vi "Send.vi"(8 "error in (no error)":errorcluster, 10 "Message":refnum<class "BaseMessage.lvclass">, 11 "StringReader in":refnum<class "StringReader.lvclass">) -> (0 "error out":errorcluster, 2 "Sent message":refnum<class "BaseMessage.lvclass">, 3 "StringReader out":refnum<class "StringReader.lvclass">)   [LabVIEW 2013, in "StringReader.lvclass"]
doc: "Send a message to the remote destination"
uses:
  StringReader.lvclass
  Message/BaseMessage/BaseMessage.lvclass
  BaseReader/BaseReader.lvclass
  <vilib>/Utility/error.llb/whitespace.ctl
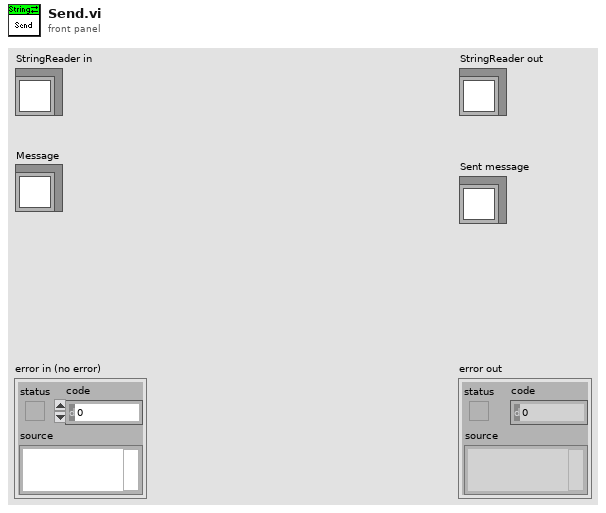
[diagram p1: front panel]
types:
  T1 = typedef "whitespace.ctl" = u16
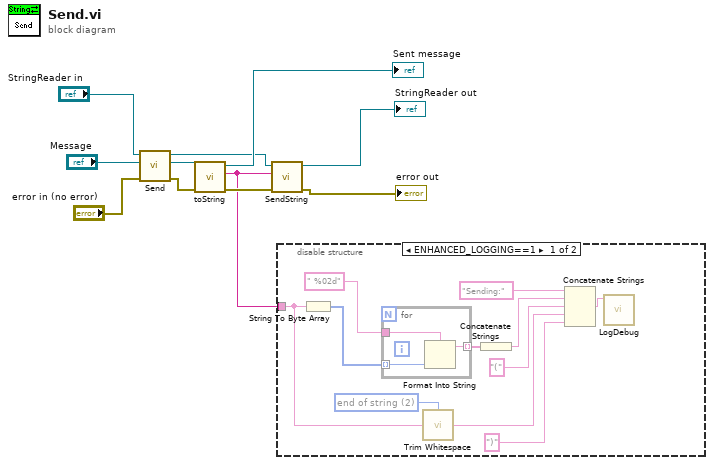
[diagram p0: block diagram]
diagram:
  n1 = call-parent "Send.vi"("error in (no error)"="error in (no error)", "Message"="Message", "BaseReader in"="StringReader in") -> ("error out"=w4:errorcluster, "Sent Message"=w7:refnum<class "BaseMessage.lvclass">, "BaseReader out"=w6:refnum<class "StringReader.lvclass">)  [unwired: 6 in]
  n2 = call-dynamic "toString.vi"("error in (no error)"=w4, "BaseMessage in"=w7) -> ("error out"=w10:errorcluster, "String"=w1:string, "BaseMessage out"=→"Sent message":refnum<class "BaseMessage.lvclass">)  [unwired: 7 in]
  n3 = call-dynamic "SendString.vi"("error in (no error)"=w10, "String"=w1, "StringReader in"=w6) -> ("error out"=→"error out":errorcluster, "StringReader out"=→"StringReader out":refnum<class "StringReader.lvclass">)  [unwired: 7 in]
  n4 = disable-structure shown="ENHANCED_LOGGING==1" {
    disable-tunnel: w1 -> [w15 _]
    frame condition #0 {
      w12 = T1 2 items=["both", "start of string", "end of string"] ("location (both)")
      n5 = String To Byte Array(string=w15) -> (unsigned byte array=w20:u8[])
      n6 = for {
        tunnel: w20 -> [w25] mode=indexing
        tunnel: [w24] -> w19 mode=indexing
        tunnel: " %02d" ("format string") -> [w23]
        n7 = Format Into String(format string=w23, w25) -> (resulting string=w24:string)  [unwired: 2 in, 1 out]
      }
      n8 = call <vilib>:"Trim Whitespace.vi"("string"=w15, "location (both)"=w12) -> ("trimmed string"=w13:string)
      n9 = Concatenate Strings(w19) -> (w18:string)
      n10 = Concatenate Strings("Sending:" ("string"), w18, "(" ("string"), w13, ")" ("string")) -> (w21:string)
      n11 = call "LogDebug.vi"("Message"=w21) -> ()  [unwired: 7 in, 1 out]
    }
    frame condition #1 (active) {
    }
  }
